vi "Gauge_Converter_FS.vi"(11 "string":string) -> (3 "decimal":i32)   [LabVIEW 2014]
uses:
  <vilib>/ptbypt/NI_PtbyPt.lvlib
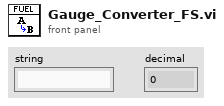
[diagram p1: front panel]
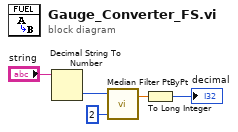
[diagram p0: block diagram]
diagram:
  n1 = Decimal String To Number(string="string") -> (number=w1:i32)  [unwired: 2 in, 1 out]
  n2 = call <vilib>:"Median Filter PtByPt.vi"("rank"=2, "x"=w1) -> ("Filtered x"=w2:dbl)  [unwired: 2 in, 1 out]
  n3 = To Long Integer(number=w2) -> (32bit integer=→"decimal":i32)
